vi "Get rake angles.vi"(7 "Circle details":T1, 10 "Edges (Falling)":T2(array[cluster]), 11 "Edges (Rising)":T2(array[cluster])) -> (2 "Falling edge angles":cluster{"Edge angles":dbl[]}[](array[cluster]), 3 "Rising edge angles":cluster{"Edge angles":dbl[]}[](array[cluster]))   [LabVIEW 2015]
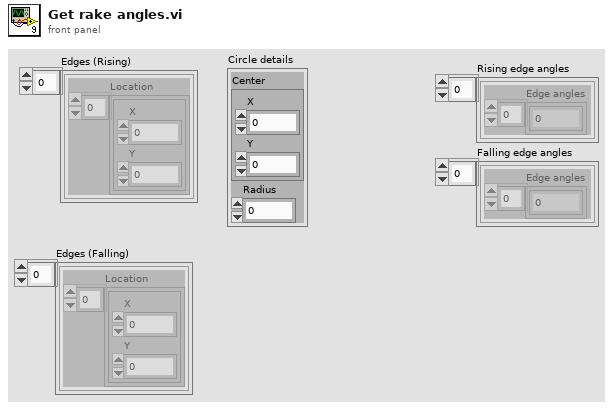
[diagram p1: front panel]
types:
  T1 = cluster{"Center":cluster{"X":sgl, "Y":sgl}, "Radius":dbl}
  T2 = cluster{"Location":cluster{"X":sgl, "Y":sgl}[]}[]
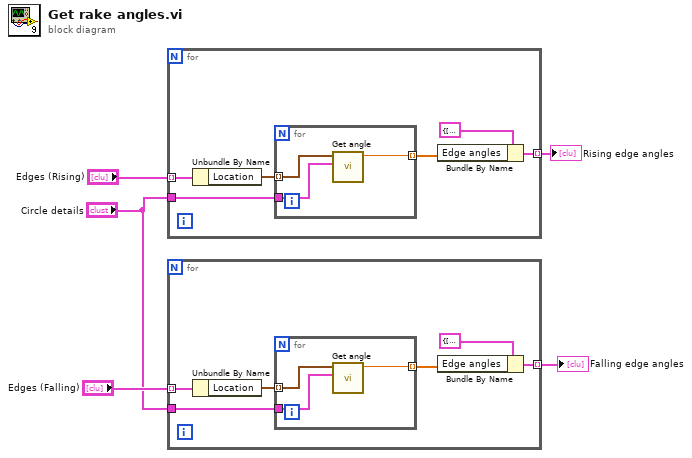
[diagram p0: block diagram]
diagram:
  n1 = for {
    tunnel: "Edges (Rising)" -> [w11] mode=indexing
    tunnel: "Circle details" -> [w9]
    tunnel: [w6] -> w4 mode=indexing
    n2 = Unbundle By Name(w11) -> ("Location"=w10:cluster{"X":sgl, "Y":sgl}[])
    n3 = for {
      tunnel: w10 -> [w14] mode=indexing
      tunnel: w9 -> [w13]
      tunnel: [w12] -> w7 mode=indexing
      n4 = call "Get angle.vi"("Circle details"=w13, "Edge location"=w14) -> ("Numeric"=w12:sgl)  [unwired: 9 in]
    }
    n5 = Bundle By Name(cluster=cluster{"Edge angles":dbl[]} {"Edge angles"=[10.123, 11.234, 12.456, 35.678, 45.987, 270.123, 355.234, 358.123]} ("Processing image rake"), "Edge angles"=w7) -> (w6:cluster{"Edge angles":dbl[]})
  }
  "Rising edge angles" <- w4
  n6 = for {
    tunnel: "Edges (Falling)" -> [w20] mode=indexing
    tunnel: "Circle details" -> [w18]
    tunnel: [w15] -> w1 mode=indexing
    n7 = Unbundle By Name(w20) -> ("Location"=w19:cluster{"X":sgl, "Y":sgl}[])
    n8 = for {
      tunnel: w19 -> [w23] mode=indexing
      tunnel: w18 -> [w22]
      tunnel: [w21] -> w16 mode=indexing
      n9 = call "Get angle.vi"("Circle details"=w22, "Edge location"=w23) -> ("Numeric"=w21:sgl)  [unwired: 9 in]
    }
    n10 = Bundle By Name(cluster=cluster{"Edge angles":dbl[]} {"Edge angles"=[10.123, 11.234, 12.456, 35.678, 45.987, 270.123, 355.234, 358.123]} ("Processing image rake"), "Edge angles"=w16) -> (w15:cluster{"Edge angles":dbl[]})
  }
  "Falling edge angles" <- w1
